vi "Get Test Params.vi"() -> ()   [LabVIEW 2025]
uses:
  19052 Example/controls/Step--numeric.ctl
panel:
  out "Instrument Info":string[](array[string])
  out "IR Parameters":T1 {"Voltage Level [V]" max=6000 format="%.3p"; "Hi Limit [ohm]" format="%#_6p"; "Lo Limit [ohm]" format="%#_6p"}
  out "DC Parameters":T2 {"Voltage Level [V]" format="%.3p"; "Hi Limit [A]" format="%#_6p"; "Lo Limit [A]" format="%#_6p"; "ARC Limit [A]" format="%#_6p"}
  out "AC Parameters":T3 {"Voltage Level [V]" format="%.3p"; "Hi Limit [A]" format="%#_6p"; "Lo Limit [A]" format="%#_6p"; "ARC Limit [A]" format="%#_6p"}
  in  "Serial Configuration":T4={"Baud Rate"=9600, "Flow Control"=0, "Parity"=0, "Data Bits"=8, "Stop Bits"=1} {"Baud Rate" items=["300"=300, "600"=600, "1200"=1200, "2400"=2400, "4800"=4800, "9600"=9600, "19200"=19200]; "Flow Control" items=["NONE", "SOFTWARE"]; "Parity" items=["NONE", "ODD", "EVEN"]; "Data Bits" items=["7"=7, "8"=8]; "Stop Bits" items=["1"=1]}
  in  "VISA resource name":refnum<visa-resource-name>="Hi-Pot_COM6"
  # "Step 1"
  # "Step 2"
  # "Step 3"
  # "19052 GET TEST \nPARAMETERS"
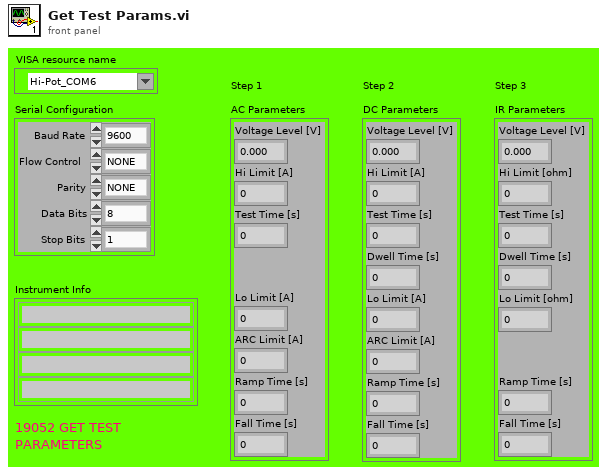
[diagram p1: front panel]
types:
  T1 = cluster{"Voltage Level [V]":u16, "Hi Limit [ohm]":dbl, "Test Time [s] ":dbl, "Dwell Time [s]":dbl, "Lo Limit [ohm]":dbl, "Ramp Time [s] ":dbl, "Fall Time [s]":dbl}
  T2 = cluster{"Voltage Level [V]":u16, "Hi Limit [A]":dbl, "Test Time [s] ":dbl, "Dwell Time [s]":dbl, "Lo Limit [A]":dbl, "ARC Limit [A]":dbl, "Ramp Time [s] ":dbl, "Fall Time [s]":dbl}
  T3 = cluster{"Voltage Level [V]":u16, "Hi Limit [A]":dbl, "Test Time [s] ":dbl, "Lo Limit [A]":dbl, "ARC Limit [A]":dbl, "Ramp Time [s] ":dbl, "Fall Time [s]":dbl}
  T4 = cluster{"Baud Rate":u32, "Flow Control":u16, "Parity":u16, "Data Bits":u16, "Stop Bits":u16}
  T5 = typedef "Step--numeric.ctl" = u8
  T6 = cluster{"Voltage Level [V] ":u16, "Hi Limit [A]":dbl, "Test Time [s] ":dbl, "Lo Limit [A]":dbl, "ARC Limit [A]":dbl, "Ramp Time [s] ":dbl, "Fall Time [s]":dbl}
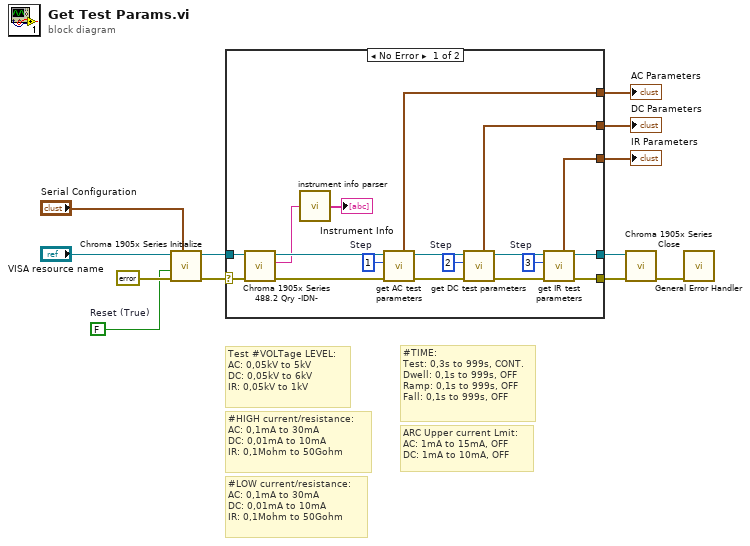
[diagram p0: block diagram]
diagram:
  w4 = FALSE  # Reset (True)
  # "ARC Upper current Lmit:\nAC: 1mA to 15mA, OFF\nDC: 1mA to 10mA, OFF"
  # "#TIME: \nTest: 0,3s to 999s, CONT. \nDwell: 0,1s to 999s, OFF\nRamp: 0,1s to 999s, OFF\nFall: 0,1s to 999s, OFF"
  # "#LOW current/resistance: \nAC: 0,1mA to 30mA\nDC: 0,01mA to 10mA\nIR: 0,1Mohm to 50Gohm"
  # "#HIGH current/resistance: \nAC: 0,1mA to 30mA\nDC: 0,01mA to 10mA\nIR: 0,1Mohm to 50Gohm"
  # "Test #VOLTage LEVEL: \nAC: 0,05kV to 5kV\nDC: 0,05kV to 6kV\nIR: 0,05kV to 1kV"
  n1 = call "Chroma 1905x Series Initialize.vi"("Serial Configuration"="Serial Configuration", "error in (no error)"=errorcluster {"status"=FALSE, "code"=0, "source"=""}, "Reset (True)"=w4, "VISA resource name"="VISA resource name") -> ("error out"=w5:errorcluster, "VISA resource name out"=w8:refnum<visa-resource-name>)  [unwired: 6 in]
  n2 = case shown="No Error" w5 {
    selector: w5 -> [w21 w32]
    tunnel: w8 -> [w20 w31]
    tunnel: [w25 w32] -> w7
    tunnel: [w24 w31] -> w6
    tunnel: [w15 _] -> w3
    tunnel: [w14 _] -> w2
    tunnel: [w13 _] -> w1
    frame No Error {
      w22 = T5 2  # Step
      w23 = T5 3  # Step
      w28 = T5 1  # Step
      n3 = call "Chroma 1905x Series 488.2 Qry -IDN-.vi"("error in (no error)"=w21, "VISA resource name"=w20) -> ("error out"=w18:errorcluster, "Result"=w17:string, "VISA resource name out"=w19:refnum<visa-resource-name>)  [unwired: 7 in]
      n4 = call "instrument info parser.vi"("ID"=w17) -> ("Instrument Info"=→"Instrument Info":string[])  [unwired: 4 in]
      n5 = call "get AC test parameters.vi"("error in (no error)"=w18, "Step"=w28, "VISA Refnum in"=w19) -> ("error out"=w30:errorcluster, "VISA Refnum out"=w29:refnum<visa-resource-name>, "AC Parameters"=w15:T6)  [unwired: 6 in]
      n6 = call "get DC test parameters.vi"("error in (no error)"=w30, "Step"=w22, "VISA Refnum in"=w29) -> ("error out"=w26:errorcluster, "VISA Refnum out"=w27:refnum<visa-resource-name>, "DC Parameters"=w14:T2)  [unwired: 6 in]
      n7 = call "get IR test parameters.vi"("error in (no error)"=w26, "Step"=w23, "VISA Refnum in"=w27) -> ("error out"=w25:errorcluster, "VISA Refnum out"=w24:refnum<visa-resource-name>, "IR Parameters"=w13:T1)  [unwired: 6 in]
    }
    frame Error {
    }
  }
  "AC Parameters" <- w3
  "DC Parameters" <- w2
  "IR Parameters" <- w1
  n8 = call "Chroma 1905x Series Close.VI"("error in (no error)"=w7, "VISA resource name"=w6) -> ("error out"=w9:errorcluster)  [unwired: 9 in]
  n9 = call <vilib>:"General Error Handler.vi"("error in (no error)"=w9) -> ()  [unwired: 10 in, 5 out]
